vi "VISA read.vi"(8 "error in (no error)":errorcluster, 11 "Cobolt in":refnum<class "Cobolt.lvclass">) -> (0 "error out":errorcluster, 2 "buffer out":string, 3 "Cobolt out":refnum<class "Cobolt.lvclass">)   [LabVIEW 2012, in "Cobolt.lvclass"]
uses:
  Cobolt.lvclass
  Cobolt.lvclass/Cobolt.ctl
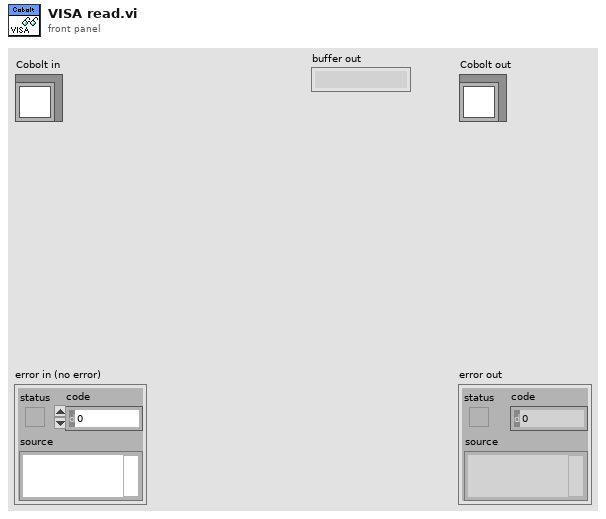
[diagram p1: front panel]
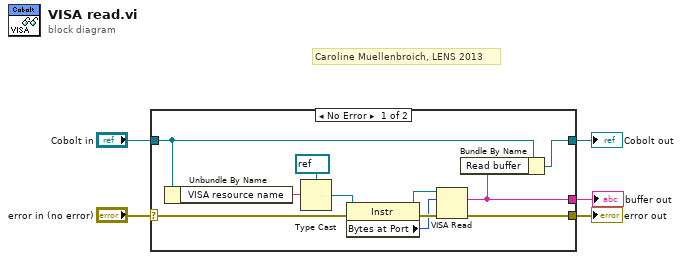
[diagram p0: block diagram]
diagram:
  # "Caroline Muellenbroich, LENS 2013"
  n1 = case shown="No Error" "error in (no error)" {
    selector: "error in (no error)" -> [w8 w18]
    tunnel: [w7 w18] -> w4
    tunnel: [w9 w17] -> w2
    tunnel: "Cobolt in" -> [w10 w17]
    tunnel: [w6 _] -> w1
    frame No Error {
      n2 = Unbundle By Name(w10) -> ("VISA resource name"=w12:string)
      n3 = Type Cast(type=refnum<visa-resource-name> refnum ("reference"), x=w12) -> (*(type *) &x=w11:refnum<visa-resource-name>)
      n4 = property class="Instr"(reference=w11, error in=w8) -> (reference out=w15:refnum<visa-resource-name>, error out=w16:errorcluster, "Bytes at Port"=w14:u32)
      n5 = VISA Read(VISA resource name=w15, byte count=w14, error in (no error)=w16) -> (read buffer=w6:string, error out=w7:errorcluster)  [unwired: 2 out]
      n6 = Bundle By Name(cluster=w10, "Read buffer"=w6) -> (w9:refnum<class "Cobolt.lvclass">)
    }
    frame Error {
    }
  }
  "error out" <- w4
  "Cobolt out" <- w2
  "buffer out" <- w1
